vi "AgilentDMM.vi"(4 "error in":T15, 7 "Command":T16) -> (0 "error out":T15, 3 "Response":T13)   [LabVIEW 2018]
uses:
  MOKO_LabViewLibrary/MokoLowLevel/MokoLowLovelControl/MLLC_Command.ctl
  MOKO_LabViewLibrary/MokoLowLevel/MokoLowLovelControl/MLLC_Error.ctl
  MOKO_LabViewLibrary/MokoLowLevel/MokoLowLovelControl/MLLC_Mode.ctl
  MOKO_LabViewLibrary/MokoLowLevel/MokoLowLovelControl/MLLC_Response.ctl
  MOKO_LabViewLibrary/MokoLowLevel/MokoLowLovelControl/MLLC_DriverName.ctl
  MOKO_LabViewLibrary/MokoLowLevel/MokoLowLovelControl/MLLC_Request.ctl
  MOKO_LabViewLibrary/MokoLowLevel/MokoLowLovelControl/MLLC_ErrorCode.ctl
  MOKO_LabViewLibrary/MokoLowLevel/MokoLowLovelControl/MLLC_ResponseInit.ctl
  MOKO_LabViewLibrary/MokoLowLevel/MokoLowLovelControl/MLLC_ConnectCluster.ctl
  MOKO_LabViewLibrary/MokoLowLevel/MokoLowLovelControl/MLLC_InterfaceType.ctl
  MOKO_LabViewLibrary/MokoLowLevel/MokoLowLovelControl/MLLC_OpenedSession.ctl
  MOKO_LabViewLibrary/MokoLowLevel/MokoLowLovelControl/MLLC_InterfaceSettings.ctl
  MOKO_LabViewLibrary/MokoLowLevel/MokoLowLovelControl/MLLC_InterfaceKind.ctl
  data/AgilentDMM_Functions.ctl
  data/AgilentDMM_Models.ctl
panel:
  in  "Settings":T9={"Saved Data"=variant, "Data"={"Connect"={"InterfaceType"=enum."VISA", "OpenedSession"="", "InterfaceSettings"={"Interface"=enum."GPIB", "EOS 4 read"=enum."LF (\\n)", "EOS 4 write"=enum."LF (\\n)", "TMO, ms"=5000, "Sett"=variant(cluster{"Baud Rate":u32, "Data Bits":u16, "Parity":u16, "Stop Bits":u16, "Flow Control":u16, "Eho":bool} {"Baud Rate"=75, "Data Bits"=0, "Parity"=0, "Stop Bits"=0, "Flow Control"=0, "Eho"=FALSE})}}, "Channel"=1, "Func"=enum."VDC", "Model"=enum."L4411"}}
  in  "Response Init array":T10[](array[typedef])=["34401", "34405", "34410", "34411", "34420", "34450", "34461", "34465", "34470", "34475", "U2741"]
  in  "Error Code":T6=5475
  in  "Request":T11="*idn?"
  in  "Driver Name":T12="AgilentDMM"
  in  "Mode":T14=enum."Check"
  # "AgilentDMM"
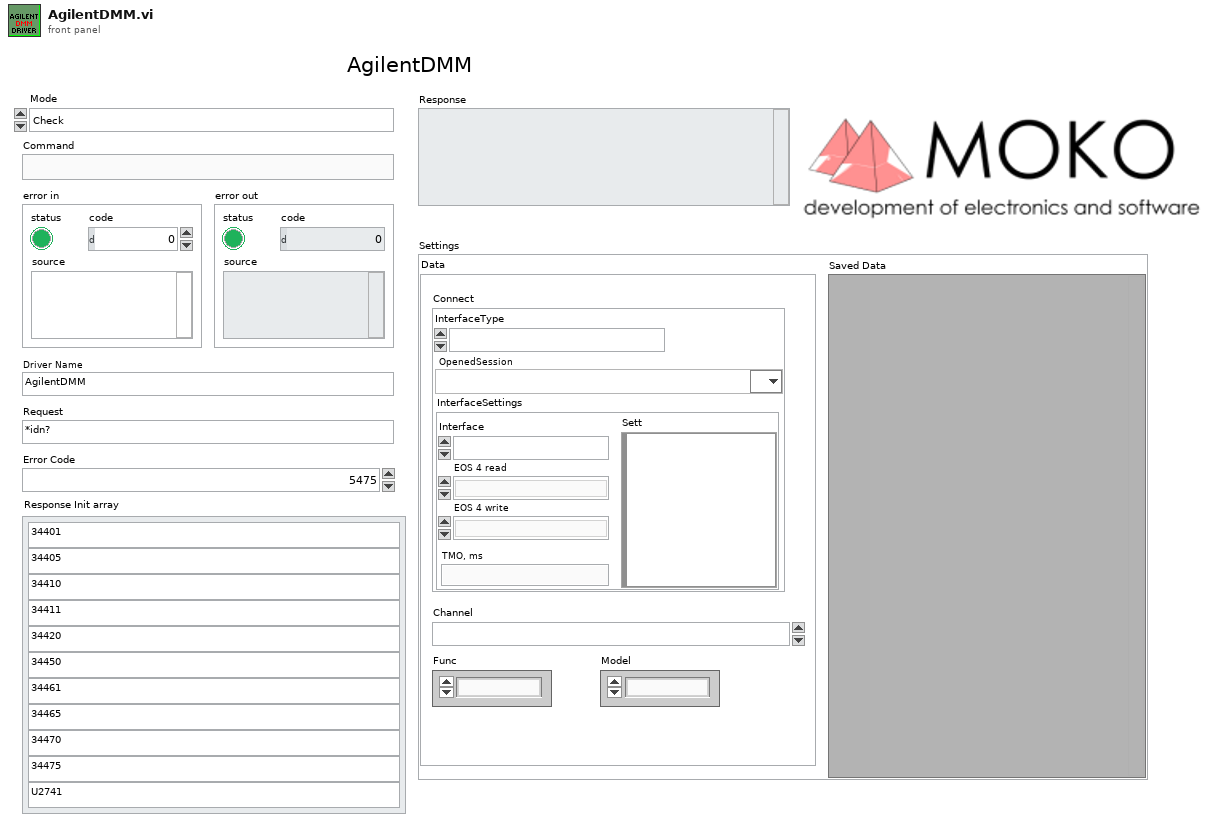
[diagram p1: front panel]
types:
  T1 = typedef "MLLC_ConnectCluster.ctl" = cluster{"InterfaceType":T2, "OpenedSession":T3, "InterfaceSettings":T4}
  T2 = typedef "MLLC_InterfaceType.ctl" = enum16{"VISA", "Prologix USB-GPIB"}
  T3 = typedef "MLLC_OpenedSession.ctl" = refnum<visa-resource-name>
  T4 = typedef "MLLC_InterfaceSettings.ctl" = cluster{"Interface":T5, "EOS 4 read":enum16{"Default (=EOS 4 write)", "CR (\\r)", "LF (\\n)", "None"}, "EOS 4 write":enum16{"CR+LF (\\r\\n)", "CR (\\r)", "LF (\\n)", "None"}, "TMO, ms":i32, "Sett":variant}
  T5 = typedef "MLLC_InterfaceKind.ctl" = enum16{"RS232", "GPIB", "USB", "Ethernet", "another"}
  T6 = typedef "MLLC_ErrorCode.ctl" = u32
  T7 = typedef "AgilentDMM_Functions.ctl" = enum16{"VDC", "VAC", "IDC", "IAC", "F", "R2", "R4", "CAP"}
  T8 = typedef "AgilentDMM_Models.ctl" = enum16{"34401", "34461", "34410", "34411", "34420", "34450", "34405", "U2741", "34470", "34465", "34460", "L4411"}
  T9 = cluster{"Saved Data":variant, "Data":cluster{"Connect":T1, "Channel":T6, "Func":T7, "Model":T8}}
  T10 = typedef "MLLC_ResponseInit.ctl" = string
  T11 = typedef "MLLC_Request.ctl" = string
  T12 = typedef "MLLC_DriverName.ctl" = string
  T13 = typedef "MLLC_Response.ctl" = string
  T14 = typedef "MLLC_Mode.ctl" = enum16{"get", "set", "close", "Init", "Check"}
  T15 = typedef "MLLC_Error.ctl" = errorcluster
  T16 = typedef "MLLC_Command.ctl" = string
  T17 = cluster{"Connect":T1, "Channel":T6, "Func":T7, "Model":T8}
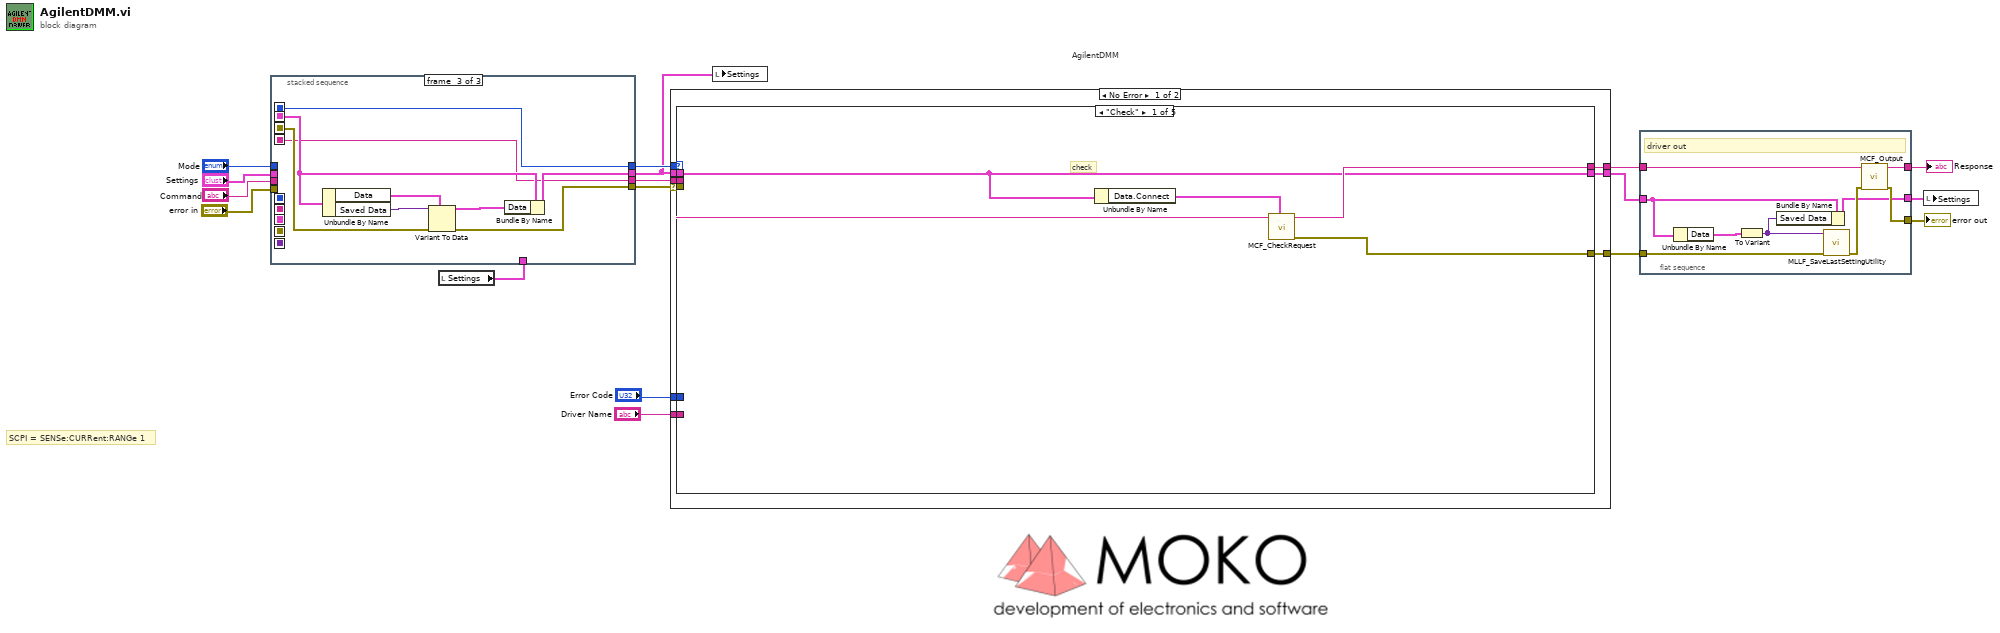
[diagram p0: block diagram]
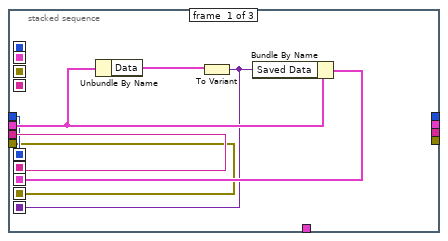
[diagram p2: hidden frame]
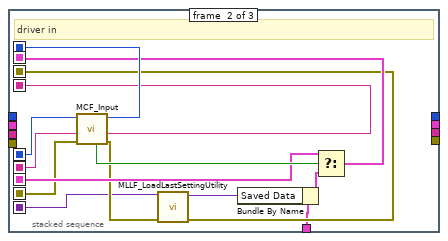
[diagram p3: hidden frame]
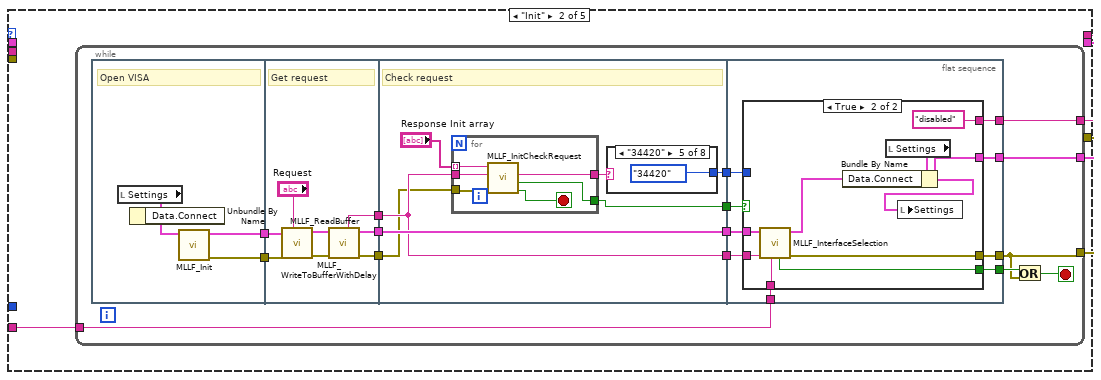
[diagram p4: hidden frame]
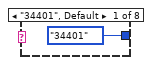
[diagram p5: hidden frame]
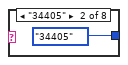
[diagram p6: hidden frame]
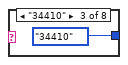
[diagram p7: hidden frame]
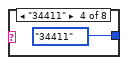
[diagram p8: hidden frame]
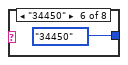
[diagram p9: hidden frame]
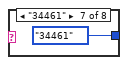
[diagram p10: hidden frame]
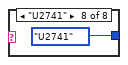
[diagram p11: hidden frame]
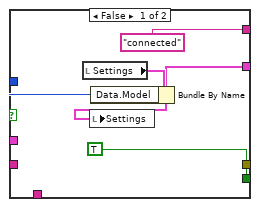
[diagram p12: hidden frame]
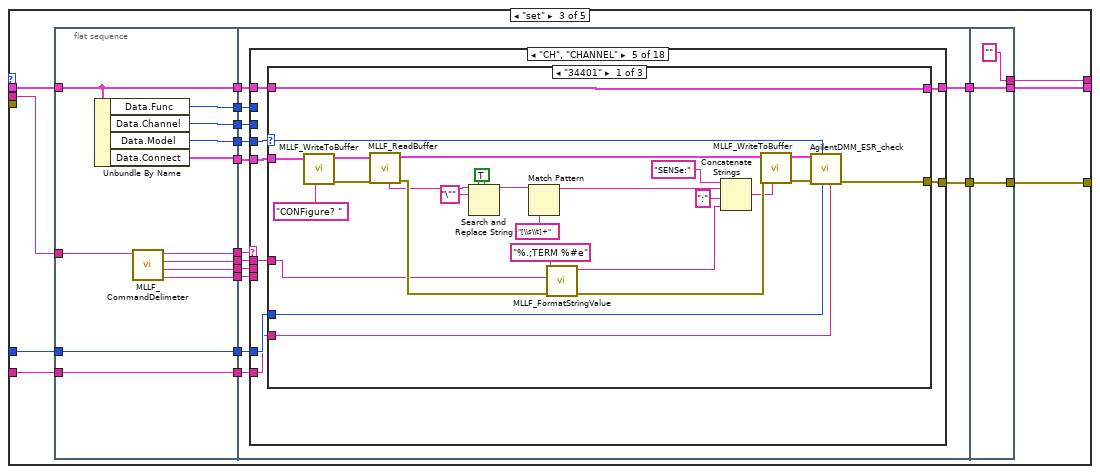
[diagram p13: hidden frame]
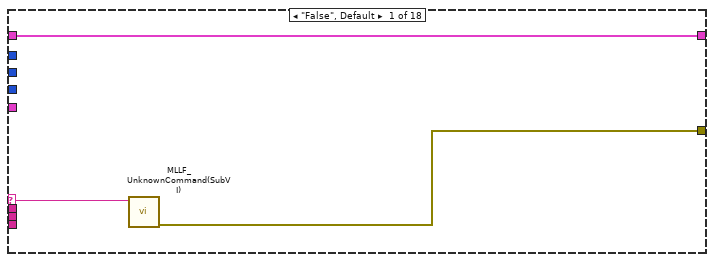
[diagram p14: hidden frame]
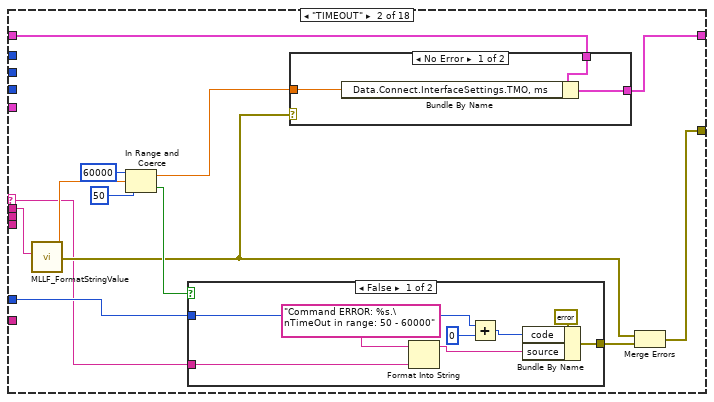
[diagram p15: hidden frame]
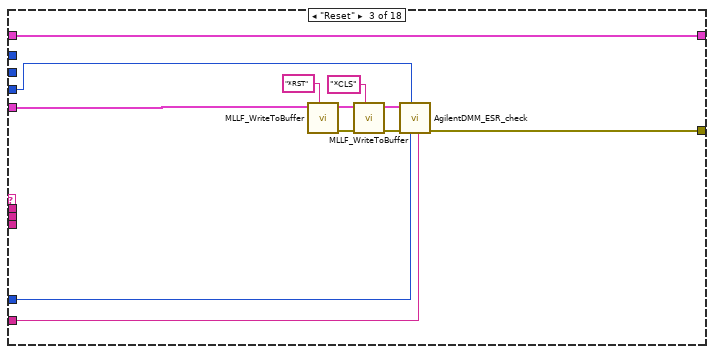
[diagram p18: hidden frame]
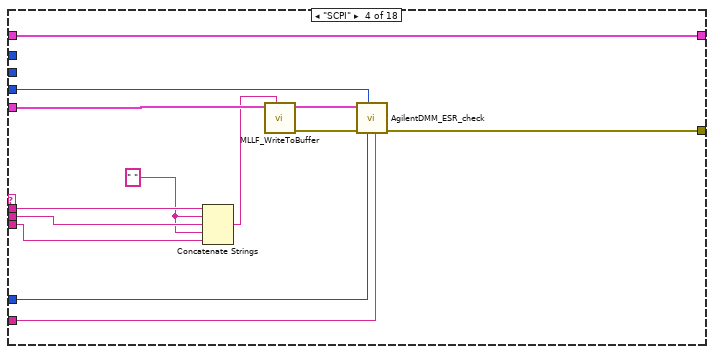
[diagram p19: hidden frame]
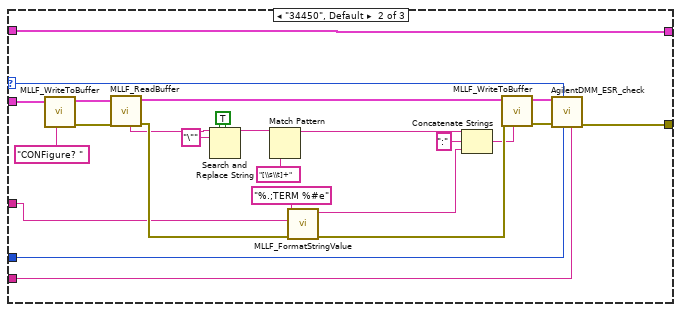
[diagram p20: hidden frame]
diagram:
  # "SCPI = SENSe:CURRent:RANGe 1"
  # "AgilentDMM"
  n1 = local read "Settings"() -> (w8:T9)
  n2 = stacked-sequence {
    seq-local: [w20 _ _] -> [_ w36 _]
    seq-local: [w19 _ _] -> [_ w37 _]
    seq-local: [w22 _ _] -> [_ w32 _]
    seq-local: [w18 _ _] -> [_ w31 _]
    seq-local: [w21 _ _] -> [_ w27 _]
    seq-local: [_ w28 _] -> [_ _ w44]
    seq-local: [_ w38 _] -> [_ _ w41]
    seq-local: [_ w35 _] -> [_ _ w40]
    seq-local: [_ w34 _] -> [_ _ w45]
    tunnel: "Command" -> [w20 _ _]
    tunnel: "Mode" -> [w19 _ _]
    tunnel: "error in" -> [w18 _ _]
    tunnel: "Settings" -> [w23 _ _]
    tunnel: w8 -> [_ w26 _]
    tunnel: [_ _ w40] -> w10
    tunnel: [_ _ w43] -> w1
    tunnel: [_ _ w42] -> w9
    tunnel: [_ _ w41] -> w11
    frame #0 {
      n3 = Unbundle By Name(w23) -> ("Data"=w24:T17)
      n4 = To Variant(anything=w24) -> (Variant=w21:variant)
      n5 = Bundle By Name(cluster=w23, "Saved Data"=w21) -> (w22:T9)
    }
    frame #1 {
      # "driver in"
      n6 = call "MCF_Input.vi"("Error In"=w31, "Command in"=w36, "Mode in"=w37) -> ("Error Out"=w30:errorcluster, "Command out"=w35:string, "Mode out"=w38:T14, "Boolean"=w33:bool)  [unwired: 5 in]
      n7 = call "MLLF_LoadLastSettingUtility.vi"("Error In"=w30, "Save data in"=w27) -> ("Error Out"=w28:errorcluster, "Save data out"=w25:variant)  [unwired: 8 in]
      n8 = Bundle By Name(cluster=w26, "Saved Data"=w25) -> (w29:T9)
      n9 = Select(t=w32, s=w33, f=w29) -> (s? t:f=w34:T9)
    }
    frame #2 {
      n10 = Unbundle By Name(w45) -> ("Data"=w46:T17, "Saved Data"=w39:variant)
      n11 = Variant To Data(error in=w44, type=w46, Variant=w39) -> (data=w47:T17, error out=w42:errorcluster)
      n12 = Bundle By Name(cluster=w45, "Data"=w47) -> (w43:T9)
    }
  }
  n13 = case shown="No Error" w9 {
    selector: w9 -> [w53 w1079]
    tunnel: [w54 w1079] -> w5
    tunnel: w11 -> [w56 _]
    tunnel: [w55 "An error occurred in the driver input module." ("String")] -> w7
    tunnel: w10 -> [w48 _]
    tunnel: w1 -> [w49 w1078]
    tunnel: "Error Code" -> [w52 _]
    tunnel: "Driver Name" -> [w51 _]
    tunnel: [w50 w1078] -> w6
    frame No Error {
      n14 = case shown="\"Check\"" w56 {
        tunnel: [w60 w65 w150 w881 "" ("String")] -> w55
        tunnel: [w61 w63 w153 w882 w1075] -> w54
        tunnel: w53 -> [_ _ _ w899 _]
        tunnel: w52 -> [_ _ w156 w901 _]
        tunnel: w51 -> [w59 w62 w154 w900 _]
        tunnel: [w58 w64 w155 w902 w1074] -> w50
        tunnel: w49 -> [w58 _ w138 w889 w1074]
        tunnel: w48 -> [_ _ w137 w888 _]
        frame "Check" {
          # "check"
          n15 = Unbundle By Name(w58) -> ("Data.Connect"=w57:T1)
          n16 = call "MCF_CheckRequest.vi"("Permanent data.Connect"=w57, "Driver Name"=w59) -> ("Error Out"=w61:errorcluster, "Output String"=w60:string)  [unwired: 8 in]
        }
        frame "Init" {
          n17 = while {
            tunnel: [w68] -> w63
            tunnel: [w67] -> w65
            tunnel: [w66] -> w64
            tunnel: w62 -> [w70]
            stop <- w80 stop-if-true
            n18 = flat-sequence {
              tunnel: [w84] -> w79
              tunnel: [w83] -> w78
              tunnel: w79 -> [w89]
              tunnel: w78 -> [w88]
              tunnel: [w87] -> w77
              tunnel: [w86] -> w76
              tunnel: [w85] -> w75
              tunnel: w77 -> [w95]
              tunnel: w76 -> [w99]
              tunnel: w75 -> [w98]
              tunnel: [w99] -> w74
              tunnel: [w98] -> w73
              tunnel: [w94] -> w72
              tunnel: [w93] -> w71
              tunnel: w74 -> [w121]
              tunnel: w73 -> [w119]
              tunnel: w72 -> [w122]
              tunnel: w71 -> [w120]
              tunnel: w70 -> [w118]
              tunnel: [w117] -> w69
              tunnel: [w116] -> w68
              tunnel: [w115] -> w67
              tunnel: [w114] -> w66
              frame #0 {
                # "Open VISA"
                n19 = local read "Settings"() -> (w82:T9)
                n20 = Unbundle By Name(w82) -> ("Data.Connect"=w81:T1)
                n21 = call "MLLF_Init.vi"("DriverConnect in"=w81) -> ("Error Out"=w84:errorcluster, "DriverConnect out"=w83:T1)  [unwired: 7 in]
              }
              frame #1 {
                # "Get request"
                n22 = call "MLLF_WriteToBufferWithDelay.vi"("Command"="Request", "Error In"=w89, "DriverConnect in"=w88) -> ("Error Out"=w91:errorcluster, "DriverConnect out"=w92:T1)  [unwired: 7 in]
                n23 = call "MLLF_ReadBuffer.vi"("Error In"=w91, "DriverConnect in"=w92) -> ("Error Out"=w87:errorcluster, "DriverConnect out"=w86:T1, "String"=w85:string)  [unwired: 6 in]
              }
              frame #2 {
                # "Check request"
                n24 = for {
                  tunnel: [w102] -> w96
                  tunnel: w98 -> [w104]
                  tunnel: "Response Init array" -> [w105] mode=indexing
                  tunnel: w95 -> [w103]
                  tunnel: [w100] -> w94
                  stop <- w101 stop-if-true
                  n25 = call "MLLF_InitCheckRequest.vi"("error in (no error)"=w103, "Answer"=w104, "Response Init"=w105) -> ("Design ARRAY STOP?"=w101:bool, "Design Interf ARRAY?"=w100:bool, "ResponseInit out"=w102:string)  [unwired: 5 in, 1 out]
                }
                n26 = case shown="\"34420\"" w96 {
                  tunnel: [AgilentDMM_Models."34401" ("Model") AgilentDMM_Models."34405" ("Model") AgilentDMM_Models."34410" ("Model") AgilentDMM_Models."34411" ("Model") AgilentDMM_Models."34420" ("Model") AgilentDMM_Models."34450" ("Model") AgilentDMM_Models."34461" ("Model") AgilentDMM_Models."U2741" ("Model")] -> w93
                  frame "34401", Default {
                  }
                  frame "34405" {
                  }
                  frame "34410" {
                  }
                  frame "34411" {
                  }
                  frame "34420" {
                  }
                  frame "34450" {
                  }
                  frame "34461" {
                  }
                  frame "U2741" {
                  }
                }
              }
              frame #3 {
                n27 = case shown="True" w122 {
                  tunnel: w121 -> [_ w135]
                  tunnel: [TRUE w130] -> w117
                  tunnel: [_ w133] -> w116
                  tunnel: w120 -> [w125 _]
                  tunnel: ["connected" "disabled"] -> w115
                  tunnel: [w123 w131] -> w114
                  tunnel: w119 -> [_ w128]
                  tunnel: w118 -> [_ w129]
                  frame False {
                    n28 = local read "Settings"() -> (w126:T9)
                    n29 = Bundle By Name(cluster=w126, "Data.Model"=w125) -> (w123:T9)
                    n30 = local write "Settings"(w123) -> ()
                  }
                  frame True {
                    n31 = call "MLLF_InterfaceSelection.vi"("Driver Name"=w129, "Answer:"=w128, "DriverConnect in"=w135) -> ("error out"=w133:T15, "DriverConnect out"=w134:T1, "stop init?"=w130:bool)  [unwired: 4 in, 2 out]
                    n32 = local read "Settings"() -> (w136:T9)
                    n33 = Bundle By Name(cluster=w136, "Data.Connect"=w134) -> (w131:T9)
                    n34 = local write "Settings"(w131) -> ()
                  }
                }
              }
            }
            n35 = Or(x=w69, y=w68) -> (x .or. y?=w80:bool)
          }
        }
        frame "set" {
          n36 = flat-sequence {
            tunnel: w154 -> [w167]
            tunnel: w138 -> [w157]
            tunnel: w156 -> [w168]
            tunnel: [w168] -> w149
            tunnel: [w157] -> w148
            tunnel: [w167] -> w147
            tunnel: [w163] -> w146
            tunnel: [w164] -> w145
            tunnel: [w165] -> w144
            tunnel: [w166] -> w143
            tunnel: [w158] -> w142
            tunnel: [w159] -> w141
            tunnel: [w160] -> w140
            tunnel: [w161] -> w139
            tunnel: w137 -> [w162]
            tunnel: [w179] -> w152
            tunnel: [w171] -> w151
            tunnel: w149 -> [w181]
            tunnel: w148 -> [w180]
            tunnel: w147 -> [w178]
            tunnel: w146 -> [w177]
            tunnel: w145 -> [w176]
            tunnel: w144 -> [w175]
            tunnel: w143 -> [w174]
            tunnel: w142 -> [w173]
            tunnel: w141 -> [w172]
            tunnel: w140 -> [w170]
            tunnel: w139 -> [w169]
            tunnel: [w879] -> w153
            tunnel: [w880] -> w155
            tunnel: w152 -> [w880]
            tunnel: w151 -> [w879]
            tunnel: ["" ("String")] -> w150
            frame #0 {
              n37 = Unbundle By Name(w157) -> ("Data.Func"=w166:T7, "Data.Channel"=w165:T6, "Data.Model"=w164:T8, "Data.Connect"=w163:T1)
              n38 = call "MLLF_CommandDelimeter.vi"("command with param"=w162) -> ("param 3"=w161:string, "param 2"=w160:string, "param 1"=w159:string, "command"=w158:string)  [unwired: 6 in, 1 out]
            }
            frame #1 {
              n39 = case shown="\"CH\", \"CHANNEL\"" w173 {
                selector: w173 -> [w183 w186 _ _ _ _ w321 _ _ _ _ _ _ w735 w796 w823 w850 w864]
                tunnel: w172 -> [_ w185 _ w226 w235 _ w322 w397 _ w474 w545 w577 w653 w736 w797 w824 w851 w865]
                tunnel: [w182 w191 w212 w231 w238 _ w328 w401 _ w478 w564 w581 w657 w740 w819 w846 w860 w871] -> w171
                tunnel: w181 -> [_ w192 w214 w233 w241 _ w330 w400 _ w477 w563 w580 w656 w737 w801 w828 w855 w873]
                tunnel: w180 -> [w184 w196 w221 w234 w242 w320 w324 w402 w472 w479 w565 w582 w658 w741 w820 w847 w861 w877]
                tunnel: [w184 w197 w221 w234 w237 w320 w323 w402 w472 w479 w565 w582 w658 w741 w820 w847 w861 w877] -> w179
                tunnel: w177 -> [_ _ w210 w229 w239 _ w327 w398 _ w475 w560 w578 w654 w739 w817 w844 w853 w869]
                tunnel: w178 -> [_ _ w213 w232 w240 _ w329 w399 _ w476 w562 w579 w655 w738 w802 w829 w856 w872]
                tunnel: w176 -> [_ _ w211 w230 w236 _ w326 w396 _ w473 w561 w576 w652 w734 w818 w845 w859 w876]
                tunnel: w175 -> [_ _ _ _ _ _ w325 _ _ _ _ _ _ _ _ _ _ _]
                tunnel: w174 -> [_ _ _ _ _ _ _ _ _ _ _ _ _ _ _ _ _ _]
                tunnel: w170 -> [_ _ _ w225 _ _ _ _ _ _ _ _ _ _ _ _ _ _]
                tunnel: w169 -> [_ _ _ w224 _ _ _ _ _ _ _ _ _ _ _ _ _ _]
                frame "False", Default {
                  n40 = call "MLLF_UnknownCommand(SubVI).vi"("Unknown command"=w183) -> ("error out"=w182:errorcluster)  [unwired: 10 in]
                }
                frame "TIMEOUT" {
                  n41 = call "MLLF_FormatStringValue.vi"("String Value"=w185) -> ("error out"=w187:T15, "number"=w188:dbl)  [unwired: 8 in, 1 out]
                  n42 = In Range and Coerce(upper limit=60000, x=w188, lower limit=50) -> (coerced(x)=w193:dbl, In Range?=w189:bool)
                  n43 = case shown="False" w189 {
                    tunnel: [w204 _] -> w190
                    tunnel: w192 -> [w203 _]
                    tunnel: w186 -> [w202 _]
                    frame False {
                      n44 = Format Into String(format string="Command ERROR: %s.\nTimeOut in range: 50 - 60000", w202) -> (resulting string=w206:string)  [unwired: 2 in, 1 out]
                      n45 = Add(x=w203, y=0) -> (x+y=w207:T6)
                      n46 = Bundle By Name(cluster=errorcluster {"status"=TRUE, "code"=0, "source"=""} ("error out"), "code"=w207, "source"=w206) -> (w204:errorcluster)
                    }
                    frame True {
                    }
                  }
                  n47 = case shown="No Error" w187 {
                    tunnel: [w200 w201] -> w197
                    tunnel: w196 -> [w199 w201]
                    tunnel: w193 -> [w198 _]
                    frame No Error {
                      n48 = Bundle By Name(cluster=w199, "Data.Connect.InterfaceSettings.TMO, ms"=w198) -> (w200:T9)
                    }
                    frame Error {
                    }
                  }
                  n49 = Merge Errors(w187, w190) -> (w191:errorcluster)
                }
                frame "Reset" {
                  n50 = call "MLLF_WriteToBuffer.vi"("String"="*RST", "DriverConnect in"=w210) -> ("error out"=w219:T15, "DriverConnect out"=w220:T1)  [unwired: 6 in]
                  n51 = call "MLLF_WriteToBuffer.vi"("String"="*CLS" ("write buffer"), "error in"=w219, "DriverConnect in"=w220) -> ("error out"=w216:T15, "DriverConnect out"=w215:T1)  [unwired: 5 in]
                  n52 = call "AgilentDMM_ESR_check.vi"("Driver Name"=w213, "Error Code"=w214, "Model"=w211, "error in"=w216, "DriverConnect in"=w215) -> ("error out"=w212:T15)  [unwired: 5 in, 1 out]
                }
                frame "SCPI" {
                  w223 = " " ("string")
                  n53 = Concatenate Strings(w226, w223, w225, w223, w224) -> (w222:string)
                  n54 = call "MLLF_WriteToBuffer.vi"("String"=w222, "DriverConnect in"=w229) -> ("error out"=w227:T15, "DriverConnect out"=w228:T1)  [unwired: 6 in]
                  n55 = call "AgilentDMM_ESR_check.vi"("Driver Name"=w232, "Error Code"=w233, "Model"=w230, "error in"=w227, "DriverConnect in"=w228) -> ("error out"=w231:T15)  [unwired: 5 in, 1 out]
                }
                frame "CH", "CHANNEL" {
                  n56 = case shown="\"34401\"" w236 {
                    selector: w236 -> [w245 w270 w296]
                    tunnel: w242 -> [w247 w272 w301]
                    tunnel: w241 -> [w249 w274 w300]
                    tunnel: w240 -> [w248 w273 w295]
                    tunnel: w239 -> [w246 w271 w299]
                    tunnel: [w250 w275 w298] -> w238
                    tunnel: [w247 w272 w297] -> w237
                    tunnel: w235 -> [w244 w269 w294]
                    frame "34401" {
                      w254 = TRUE ("replace all? (F)")
                      n57 = call "MLLF_WriteToBuffer.vi"("String"="CONFigure? ", "DriverConnect in"=w246) -> ("error out"=w263:T15, "DriverConnect out"=w264:T1)  [unwired: 6 in]
                      n58 = call "MLLF_ReadBuffer.vi"("Error In"=w263, "DriverConnect in"=w264) -> ("Error Out"=w262:errorcluster, "DriverConnect out"=w261:T1, "String"=w256:string)  [unwired: 6 in]
                      n59 = Search and Replace String(replace all?=w254, case sensitive?=w254, input string=w256, search string="\"") -> (result string=w255:string)  [unwired: 4 in, 3 out]
                      n60 = Match Pattern(string=w255, regular expression="[\\s\\t]+") -> (before substring=w257:string)  [unwired: 1 in, 3 out]
                      n61 = call "MLLF_FormatStringValue.vi"("error in"=w262, "String Value"=w244, "Format"="%.;TERM %#e" ("format string")) -> ("error out"=w268:T15, "String Value Formated"=w259:T16)  [unwired: 6 in, 1 out]
                      n62 = Concatenate Strings("SENSe:" ("string"), w257, ":" ("string"), w259) -> (w252:string)
                      n63 = call "MLLF_WriteToBuffer.vi"("String"=w252, "error in"=w268, "DriverConnect in"=w261) -> ("error out"=w267:T15, "DriverConnect out"=w266:T1)  [unwired: 5 in]
                      n64 = call "AgilentDMM_ESR_check.vi"("Driver Name"=w248, "Error Code"=w249, "Model"=w245, "error in"=w267, "DriverConnect in"=w266) -> ("error out"=w250:T15)  [unwired: 5 in, 1 out]
                    }
                    frame "34450", Default {
                      w279 = TRUE ("replace all? (F)")
                      n65 = call "MLLF_WriteToBuffer.vi"("String"="CONFigure? ", "DriverConnect in"=w271) -> ("error out"=w288:T15, "DriverConnect out"=w289:T1)  [unwired: 6 in]
                      n66 = call "MLLF_ReadBuffer.vi"("Error In"=w288, "DriverConnect in"=w289) -> ("Error Out"=w287:errorcluster, "DriverConnect out"=w286:T1, "String"=w281:string)  [unwired: 6 in]
                      n67 = Search and Replace String(replace all?=w279, case sensitive?=w279, input string=w281, search string="\"") -> (result string=w280:string)  [unwired: 4 in, 3 out]
                      n68 = Match Pattern(string=w280, regular expression="[\\s\\t]+") -> (before substring=w282:string)  [unwired: 1 in, 3 out]
                      n69 = call "MLLF_FormatStringValue.vi"("error in"=w287, "String Value"=w269, "Format"="%.;TERM %#e" ("format string")) -> ("error out"=w293:T15, "String Value Formated"=w284:T16)  [unwired: 6 in, 1 out]
                      n70 = Concatenate Strings(w282, ":" ("string"), w284) -> (w277:string)
                      n71 = call "MLLF_WriteToBuffer.vi"("String"=w277, "error in"=w293, "DriverConnect in"=w286) -> ("error out"=w292:T15, "DriverConnect out"=w291:T1)  [unwired: 5 in]
                      n72 = call "AgilentDMM_ESR_check.vi"("Driver Name"=w273, "Error Code"=w274, "Model"=w270, "error in"=w292, "DriverConnect in"=w291) -> ("error out"=w275:T15)  [unwired: 5 in, 1 out]
                    }
                    frame "34420" {
                      n73 = call "MLLF_FormatStringValue.vi"("String Value"=w294, "Format"="%d" ("format")) -> ("error out"=w313:T15, "String Value Formated"=w306:T16)  [unwired: 7 in, 1 out]
                      n74 = call "MLLF_ParameterSelect.vi"("Command to equipment"=string[] ["1", "2"] ("Parameters"), "Names"=string[][] [["1"], ["2"]], "Input"=w306, "Error In"=w313, "Command"=w294, "Driver Name"=w295, "Error Code"=w300) -> ("Choice"=w303:string, "Error Out"=w305:errorcluster)  [unwired: 7 in]
                      n75 = call "MLLF_ParameterSelect.vi"("Command to equipment"=string[] ["ROUTe:TERMinals FRONt1", "ROUTe:TERMinals FRONt2"] ("Names"), "Names"=string[][] [["1"], ["2"]], "Input"=w306, "Error In"=w305, "Command"=w294, "Driver Name"=w295, "Error Code"=w300) -> ("Choice"=w309:string, "Error Out"=w308:errorcluster)  [unwired: 7 in]
                      n76 = call "MLLF_WriteToBuffer.vi"("String"=w309, "error in"=w308, "DriverConnect in"=w299) -> ("error out"=w304:T15, "DriverConnect out"=w307:T1)  [unwired: 5 in]
                      n77 = call "AgilentDMM_ESR_check.vi"("Driver Name"=w295, "Error Code"=w300, "Model"=w296, "error in"=w304, "DriverConnect in"=w307) -> ("error out"=w298:T15)  [unwired: 5 in, 1 out]
                      n78 = Decimal String To Number(string=w303) -> (number=w302:i32)  [unwired: 2 in, 1 out]
                      n79 = case shown="No Error" w298 {
                        tunnel: [w318 w319] -> w297
                        tunnel: w301 -> [w317 w319]
                        tunnel: w302 -> [w316 _]
                        frame No Error {
                          n80 = Bundle By Name(cluster=w317, "Data.Channel"=w316) -> (w318:T9)
                        }
                        frame Error {
                        }
                      }
                    }
                  }
                }
                frame "<----MAIN FUNCTIONS---->" {
                }
                frame "Func", "Function" {
                  # "FUNC=VDC"
                  n81 = case shown="Default" w326 {
                    selector: w326 -> [w357 w379]
                    tunnel: w322 -> [w356 w368]
                    tunnel: w330 -> [w363 w383]
                    tunnel: w329 -> [w362 w382]
                    tunnel: [w361 w381] -> w328
                    tunnel: w327 -> [w359 w380]
                    tunnel: w325 -> [_ w374]
                    tunnel: w321 -> [w355 _]
                    frame Default {
                      n82 = call "MLLF_ParameterSelect.vi"("Command to equipment"=string[] ["CONF:VOLT:DC auto", "CONF:VOLT:AC auto", "CONF:CURR:DC auto", "CONF:CURR:AC auto", "CONF:RES auto", "CONF:FRES auto", "CONF:FREQ", "CONF:TC", "CONF:PER", "CONF:TEMP", "CONF:CAP auto"] ("Names"), "Names"=string[][] [["VDC", "", ""], ["VAC", "", ""], ["IDC", "", ""], ["IAC", "", ""], ["R", "R2", "R2WIRE"], ["R4", "R4WIRE", ""], ["F", "", ""], ["TC", "", ""], ["P", "Period", ""], ["RTD", "PRT", ""], ["C", "CAP", ""]], "Input"=w356, "Command"=w355, "Driver Name"=w362, "Error Code"=w363) -> ("Choice"=w358:string, "Error Out"=w360:errorcluster)  [unwired: 8 in]
                      n83 = call "MLLF_WriteToBuffer.vi"("String"=w358, "error in"=w360, "DriverConnect in"=w359) -> ("error out"=w367:T15, "DriverConnect out"=w366:T1)  [unwired: 5 in]
                      n84 = call "AgilentDMM_ESR_check.vi"("Driver Name"=w362, "Error Code"=w363, "Model"=w357, "error in"=w367, "DriverConnect in"=w366) -> ("error out"=w361:T15)  [unwired: 5 in, 1 out]
                    }
                    frame "34420" {
                      n85 = Equal?(x=u8 1 ("y"), y=w374) -> (x = y?=w376:bool)
                      n86 = Select(t="ROUTe:TERMinals FRONt1" ("String"), s=w376, f="ROUTe:TERMinals FRONt2" ("String")) -> (s? t:f=w370:string)
                      n87 = call "MLLF_ParameterSelect.vi"("Command to equipment"=string[] ["CONF:VOLT:DC auto", "CONF:RES auto", "CONF:FRES auto", "CONF:TC", "CONF:TEMP"] ("Names"), "Names"=string[][] [["VDC", "", ""], ["R", "R2", "R2WIRE"], ["R4", "R4WIRE", ""], ["TC", "", ""], ["RTD", "PRT", ""]], "Input"=w368, "Command"=w368, "Driver Name"=w382, "Error Code"=w383) -> ("Choice"=w369:string, "Error Out"=w371:errorcluster)  [unwired: 8 in]
                      n88 = case shown="\"True\", Default" w369 {
                        selector: w369 -> [w388 w390]
                        tunnel: [w388 w394] -> w373
                        tunnel: [w389 w393] -> w372
                        tunnel: w371 -> [w389 w392]
                        tunnel: w370 -> [_ w391]
                        frame "False" {
                        }
                        frame "True", Default {
                          n89 = Format Into String(format string="%S\n%S", error in=w392, w390, w391) -> (resulting string=w394:string, error out=w393:errorcluster)  [unwired: 1 in]
                        }
                      }
                      n90 = call "MLLF_WriteToBuffer.vi"("String"=w373, "error in"=w372, "DriverConnect in"=w380) -> ("error out"=w387:T15, "DriverConnect out"=w386:T1)  [unwired: 5 in]
                      n91 = call "AgilentDMM_ESR_check.vi"("Driver Name"=w382, "Error Code"=w383, "Model"=w379, "error in"=w387, "DriverConnect in"=w386) -> ("error out"=w381:T15)  [unwired: 5 in, 1 out]
                    }
                  }
                  n92 = case shown="\"IDC\"" w322 {
                    tunnel: w324 -> [w333 w336 w339 w342 w345 w348 w351 w354]
                    tunnel: [w332 w335 w338 w341 w344 w347 w350 w353] -> w323
                    frame "VDC", Default {
                      n93 = Bundle By Name(cluster=w333, "Data.Func"=AgilentDMM_Functions."VDC" ("Func")) -> (w332:T9)
                    }
                    frame "VAC" {
                      n94 = Bundle By Name(cluster=w336, "Data.Func"=AgilentDMM_Functions."VAC" ("Func")) -> (w335:T9)
                    }
                    frame "IDC" {
                      n95 = Bundle By Name(cluster=w339, "Data.Func"=AgilentDMM_Functions."IDC" ("Func")) -> (w338:T9)
                    }
                    frame "IAC" {
                      n96 = Bundle By Name(cluster=w342, "Data.Func"=AgilentDMM_Functions."IAC" ("Func")) -> (w341:T9)
                    }
                    frame "R", "R2", "R2WI" {
                      n97 = Bundle By Name(cluster=w345, "Data.Func"=AgilentDMM_Functions."R2" ("Func")) -> (w344:T9)
                    }
                    frame "R4", "R4WI" {
                      n98 = Bundle By Name(cluster=w348, "Data.Func"=AgilentDMM_Functions."R4" ("Func")) -> (w347:T9)
                    }
                    frame "F" {
                      n99 = Bundle By Name(cluster=w351, "Data.Func"=AgilentDMM_Functions."F" ("Func")) -> (w350:T9)
                    }
                    frame "C", "CAP" {
                      n100 = Bundle By Name(cluster=w354, "Data.Func"=AgilentDMM_Functions."CAP" ("Func")) -> (w353:T9)
                    }
                  }
                }
                frame "Range" {
                  n101 = case shown="\"34401\"" w396 {
                    tunnel: [w422 w457] -> w401
                    tunnel: w400 -> [w421 w456]
                    tunnel: w399 -> [w420 w455]
                    tunnel: w396 -> [w419 w454]
                    tunnel: w398 -> [w418 w453]
                    tunnel: w397 -> [w404 w439]
                    frame "34461", Default {
                      w407 = TRUE ("replace all? (F)")
                      n102 = call "MLLF_WriteToBuffer.vi"("String"="CONFigure? ", "DriverConnect in"=w418) -> ("error out"=w415:T15, "DriverConnect out"=w416:T1)  [unwired: 6 in]
                      n103 = call "MLLF_ReadBuffer.vi"("Error In"=w415, "DriverConnect in"=w416) -> ("Error Out"=w403:errorcluster, "DriverConnect out"=w414:T1, "String"=w409:string)  [unwired: 6 in]
                      n104 = Search and Replace String(replace all?=w407, case sensitive?=w407, input string=w409, search string="\"") -> (result string=w408:string)  [unwired: 4 in, 3 out]
                      n105 = case shown="\"MIN\"" w404 {
                        selector: w404 -> [w427 _ _ _]
                        tunnel: [w430 w431 w433 w435] -> w425
                        tunnel: [w429 "RANG:AUTO ON" ("String") "RANG MIN" ("String") "RANG MAX" ("String")] -> w412
                        tunnel: w403 -> [w426 w431 w433 w435]
                        frame "False", Default {
                          n106 = call "MLLF_FormatStringValue.vi"("error in"=w426, "String Value"=w427, "Format"="RANG %#e" ("format string")) -> ("error out"=w430:T15, "String Value Formated"=w429:T16)  [unwired: 6 in, 1 out]
                        }
                        frame "Auto" {
                        }
                        frame "MIN" {
                        }
                        frame "MAX" {
                        }
                      }
                      n107 = Match Pattern(string=w408, regular expression="[\\s\\t]+") -> (before substring=w410:string)  [unwired: 1 in, 3 out]
                      n108 = Concatenate Strings(w410, ":" ("string"), w412) -> (w405:string)
                      n109 = call "MLLF_WriteToBuffer.vi"("String"=w405, "error in"=w425, "DriverConnect in"=w414) -> ("error out"=w424:T15, "DriverConnect out"=w423:T1)  [unwired: 5 in]
                      n110 = call "AgilentDMM_ESR_check.vi"("Driver Name"=w420, "Error Code"=w421, "Model"=w419, "error in"=w424, "DriverConnect in"=w423) -> ("error out"=w422:T15)  [unwired: 5 in, 1 out]
                    }
                    frame "34401" {
                      w442 = TRUE ("replace all? (F)")
                      n111 = call "MLLF_WriteToBuffer.vi"("String"="CONFigure? ", "DriverConnect in"=w453) -> ("error out"=w450:T15, "DriverConnect out"=w451:T1)  [unwired: 6 in]
                      n112 = call "MLLF_ReadBuffer.vi"("Error In"=w450, "DriverConnect in"=w451) -> ("Error Out"=w438:errorcluster, "DriverConnect out"=w449:T1, "String"=w444:string)  [unwired: 6 in]
                      n113 = Search and Replace String(replace all?=w442, case sensitive?=w442, input string=w444, search string="\"") -> (result string=w443:string)  [unwired: 4 in, 3 out]
                      n114 = case shown="\"MIN\"" w439 {
                        selector: w439 -> [w462 _ _ _]
                        tunnel: [w465 w466 w468 w470] -> w460
                        tunnel: [w464 "RANG:AUTO ON" ("String") "RANG MIN" ("String") "RANG MAX" ("String")] -> w447
                        tunnel: w438 -> [w461 w466 w468 w470]
                        frame "False", Default {
                          n115 = call "MLLF_FormatStringValue.vi"("error in"=w461, "String Value"=w462, "Format"="RANG %#e" ("format string")) -> ("error out"=w465:T15, "String Value Formated"=w464:T16)  [unwired: 6 in, 1 out]
                        }
                        frame "Auto" {
                        }
                        frame "MIN" {
                        }
                        frame "MAX" {
                        }
                      }
                      n116 = Match Pattern(string=w443, regular expression="[\\s\\t]+") -> (before substring=w445:string)  [unwired: 1 in, 3 out]
                      n117 = Concatenate Strings("SENSe:" ("string"), w445, ":" ("string"), w447) -> (w440:string)
                      n118 = call "MLLF_WriteToBuffer.vi"("String"=w440, "error in"=w460, "DriverConnect in"=w449) -> ("error out"=w459:T15, "DriverConnect out"=w458:T1)  [unwired: 5 in]
                      n119 = call "AgilentDMM_ESR_check.vi"("Driver Name"=w455, "Error Code"=w456, "Model"=w454, "error in"=w459, "DriverConnect in"=w458) -> ("error out"=w457:T15)  [unwired: 5 in, 1 out]
                    }
                  }
                }
                frame "---------ADDITIONAL---------" {
                }
                frame "Res", "Resolution" {
                  n120 = case shown="\"34401\"" w473 {
                    selector: w473 -> [w480 w513]
                    tunnel: [w499 w532] -> w478
                    tunnel: w477 -> [w498 w531]
                    tunnel: w476 -> [w497 w530]
                    tunnel: w475 -> [w496 w529]
                    tunnel: w474 -> [w481 w514]
                    frame "34461", Default {
                      w484 = TRUE ("replace all? (F)")
                      n121 = call "MLLF_WriteToBuffer.vi"("String"="CONFigure? ", "DriverConnect in"=w496) -> ("error out"=w493:T15, "DriverConnect out"=w494:T1)  [unwired: 6 in]
                      n122 = call "MLLF_ReadBuffer.vi"("Error In"=w493, "DriverConnect in"=w494) -> ("Error Out"=w492:errorcluster, "DriverConnect out"=w491:T1, "String"=w486:string)  [unwired: 6 in]
                      n123 = Search and Replace String(replace all?=w484, case sensitive?=w484, input string=w486, search string="\"") -> (result string=w485:string)  [unwired: 4 in, 3 out]
                      n124 = case shown="\"MAX\"" w481 {
                        selector: w481 -> [w504 _ _]
                        tunnel: [w507 w508 w510] -> w502
                        tunnel: [w506 "RES MAX" ("String") "RES MIN" ("String")] -> w489
                        tunnel: w492 -> [w503 w508 w510]
                        frame "False", Default {
                          n125 = call "MLLF_FormatStringValue.vi"("error in"=w503, "String Value"=w504, "Format"="RES %#e" ("format string")) -> ("error out"=w507:T15, "String Value Formated"=w506:T16)  [unwired: 6 in, 1 out]
                        }
                        frame "MAX" {
                        }
                        frame "MIN" {
                        }
                      }
                      n126 = Match Pattern(string=w485, regular expression="[\\s\\t]+") -> (before substring=w487:string)  [unwired: 1 in, 3 out]
                      n127 = Concatenate Strings(w487, ":" ("string"), w489) -> (w482:string)
                      n128 = call "MLLF_WriteToBuffer.vi"("String"=w482, "error in"=w502, "DriverConnect in"=w491) -> ("error out"=w501:T15, "DriverConnect out"=w500:T1)  [unwired: 5 in]
                      n129 = call "AgilentDMM_ESR_check.vi"("Driver Name"=w497, "Error Code"=w498, "Model"=w480, "error in"=w501, "DriverConnect in"=w500) -> ("error out"=w499:T15)  [unwired: 5 in, 1 out]
                    }
                    frame "34401" {
                      w517 = TRUE ("replace all? (F)")
                      n130 = call "MLLF_WriteToBuffer.vi"("String"="CONFigure? ", "DriverConnect in"=w529) -> ("error out"=w526:T15, "DriverConnect out"=w527:T1)  [unwired: 6 in]
                      n131 = call "MLLF_ReadBuffer.vi"("Error In"=w526, "DriverConnect in"=w527) -> ("Error Out"=w525:errorcluster, "DriverConnect out"=w524:T1, "String"=w519:string)  [unwired: 6 in]
                      n132 = Search and Replace String(replace all?=w517, case sensitive?=w517, input string=w519, search string="\"") -> (result string=w518:string)  [unwired: 4 in, 3 out]
                      n133 = case shown="\"MIN\"" w514 {
                        selector: w514 -> [w537 _ _]
                        tunnel: [w540 w541 w543] -> w535
                        tunnel: [w539 "RES MAX" ("String") "RES MIN" ("String")] -> w522
                        tunnel: w525 -> [w536 w541 w543]
                        frame "False", Default {
                          n134 = call "MLLF_FormatStringValue.vi"("error in"=w536, "String Value"=w537, "Format"="RES %#e" ("format string")) -> ("error out"=w540:T15, "String Value Formated"=w539:T16)  [unwired: 6 in, 1 out]
                        }
                        frame "MAX" {
                        }
                        frame "MIN" {
                        }
                      }
                      n135 = Match Pattern(string=w518, regular expression="[\\s\\t]+") -> (before substring=w520:string)  [unwired: 1 in, 3 out]
                      n136 = Concatenate Strings("SENSe:" ("string"), w520, ":" ("string"), w522) -> (w515:string)
                      n137 = call "MLLF_WriteToBuffer.vi"("String"=w515, "error in"=w535, "DriverConnect in"=w524) -> ("error out"=w534:T15, "DriverConnect out"=w533:T1)  [unwired: 5 in]
                      n138 = call "AgilentDMM_ESR_check.vi"("Driver Name"=w530, "Error Code"=w531, "Model"=w513, "error in"=w534, "DriverConnect in"=w533) -> ("error out"=w532:T15)  [unwired: 5 in, 1 out]
                    }
                  }
                }
                frame "Aper", "Aperture", "MeasTime" {
                  w548 = TRUE ("replace all? (F)")
                  n139 = call "MLLF_WriteToBuffer.vi"("String"="CONFigure? ", "DriverConnect in"=w560) -> ("error out"=w557:T15, "DriverConnect out"=w558:T1)  [unwired: 6 in]
                  n140 = call "MLLF_ReadBuffer.vi"("Error In"=w557, "DriverConnect in"=w558) -> ("Error Out"=w556:errorcluster, "DriverConnect out"=w555:T1, "String"=w550:string)  [unwired: 6 in]
                  n141 = Search and Replace String(replace all?=w548, case sensitive?=w548, input string=w550, search string="\"") -> (result string=w549:string)  [unwired: 4 in, 3 out]
                  n142 = case shown="\"OFF\"" w545 {
                    selector: w545 -> [w570 _]
                    tunnel: [w573 w574] -> w568
                    tunnel: [w572 "APER:ENAB OFF" ("String")] -> w553
                    tunnel: w556 -> [w569 w574]
                    frame "False", Default {
                      n143 = call "MLLF_FormatStringValue.vi"("error in"=w569, "String Value"=w570, "Format"="APER %#e" ("format string")) -> ("error out"=w573:T15, "String Value Formated"=w572:T16)  [unwired: 6 in, 1 out]
                    }
                    frame "OFF" {
                    }
                  }
                  n144 = Match Pattern(string=w549, regular expression="[\\s\\t]+") -> (before substring=w551:string)  [unwired: 1 in, 3 out]
                  n145 = Concatenate Strings(w551, ":" ("string"), w553) -> (w546:string)
                  n146 = call "MLLF_WriteToBuffer.vi"("String"=w546, "error in"=w568, "DriverConnect in"=w555) -> ("error out"=w567:T15, "DriverConnect out"=w566:T1)  [unwired: 5 in]
                  n147 = call "AgilentDMM_ESR_check.vi"("Driver Name"=w562, "Error Code"=w563, "Model"=w561, "error in"=w567, "DriverConnect in"=w566) -> ("error out"=w564:T15)  [unwired: 5 in, 1 out]
                }
                frame "IntegrationTime", "IntTime", "NPLC" {
                  n148 = case shown="\"34401\"" w576 {
                    tunnel: [w602 w636] -> w581
                    tunnel: w580 -> [w601 w635]
                    tunnel: w579 -> [w600 w634]
                    tunnel: w576 -> [w599 w633]
                    tunnel: w578 -> [w598 w632]
                    tunnel: w577 -> [w584 w618]
                    frame "34401" {
                      w587 = TRUE ("replace all? (F)")
                      n149 = call "MLLF_WriteToBuffer.vi"("String"="CONFigure? ", "DriverConnect in"=w598) -> ("error out"=w595:T15, "DriverConnect out"=w596:T1)  [unwired: 6 in]
                      n150 = call "MLLF_ReadBuffer.vi"("Error In"=w595, "DriverConnect in"=w596) -> ("DriverConnect out"=w594:T1, "String"=w589:string)  [unwired: 6 in, 1 out]
                      n151 = Search and Replace String(replace all?=w587, case sensitive?=w587, input string=w589, search string="\"") -> (result string=w588:string)  [unwired: 4 in, 3 out]
                      n152 = case shown="\"MIN\"" w584 {
                        tunnel: [w609 w613 w617] -> w605
                        tunnel: [w608 w612 w616] -> w592
                        tunnel: w584 -> [w606 w610 w614]
                        frame Default {
                          n153 = call "MLLF_FormatStringValue.vi"("String Value"=w606, "Format"="NPLC %#e" ("format string")) -> ("error out"=w609:T15, "String Value Formated"=w608:T16)  [unwired: 7 in, 1 out]
                        }
                        frame "MIN" {
                          n154 = call "MLLF_FormatStringValue.vi"("String Value"=w610, "Format"="NPLC MIN" ("format string")) -> ("error out"=w613:T15, "String Value Formated"=w612:T16)  [unwired: 7 in, 1 out]
                        }
                        frame "MAX" {
                          n155 = call "MLLF_FormatStringValue.vi"("String Value"=w614, "Format"="NPLC MAX" ("format string")) -> ("error out"=w617:T15, "String Value Formated"=w616:T16)  [unwired: 7 in, 1 out]
                        }
                      }
                      n156 = Match Pattern(string=w588, regular expression="[\\s\\t]+") -> (before substring=w590:string)  [unwired: 1 in, 3 out]
                      n157 = Concatenate Strings("SENSe:" ("string"), w590, ":" ("string"), w592) -> (w585:string)
                      n158 = call "MLLF_WriteToBuffer.vi"("String"=w585, "error in"=w605, "DriverConnect in"=w594) -> ("error out"=w604:T15, "DriverConnect out"=w603:T1)  [unwired: 5 in]
                      n159 = call "AgilentDMM_ESR_check.vi"("Driver Name"=w600, "Error Code"=w601, "Model"=w599, "error in"=w604, "DriverConnect in"=w603) -> ("error out"=w602:T15)  [unwired: 5 in, 1 out]
                    }
                    frame Default {
                      w621 = TRUE ("replace all? (F)")
                      n160 = call "MLLF_WriteToBuffer.vi"("String"="CONFigure? ", "DriverConnect in"=w632) -> ("error out"=w629:T15, "DriverConnect out"=w630:T1)  [unwired: 6 in]
                      n161 = call "MLLF_ReadBuffer.vi"("Error In"=w629, "DriverConnect in"=w630) -> ("DriverConnect out"=w628:T1, "String"=w623:string)  [unwired: 6 in, 1 out]
                      n162 = Search and Replace String(replace all?=w621, case sensitive?=w621, input string=w623, search string="\"") -> (result string=w622:string)  [unwired: 4 in, 3 out]
                      n163 = case shown="Default" w618 {
                        tunnel: [w643 w647 w651] -> w639
                        tunnel: [w642 w646 w650] -> w626
                        tunnel: w618 -> [w640 w644 w648]
                        frame Default {
                          n164 = call "MLLF_FormatStringValue.vi"("String Value"=w640, "Format"="%.;NPLC %#e" ("format string")) -> ("error out"=w643:T15, "String Value Formated"=w642:T16)  [unwired: 7 in, 1 out]
                        }
                        frame "MIN" {
                          n165 = call "MLLF_FormatStringValue.vi"("String Value"=w644, "Format"="NPLC MIN" ("format string")) -> ("error out"=w647:T15, "String Value Formated"=w646:T16)  [unwired: 7 in, 1 out]
                        }
                        frame "MAX" {
                          n166 = call "MLLF_FormatStringValue.vi"("String Value"=w648, "Format"="NPLC MAX" ("format string")) -> ("error out"=w651:T15, "String Value Formated"=w650:T16)  [unwired: 7 in, 1 out]
                        }
                      }
                      n167 = Match Pattern(string=w622, regular expression="[\\s\\t]+") -> (before substring=w624:string)  [unwired: 1 in, 3 out]
                      n168 = Concatenate Strings(w624, ":" ("string"), w626) -> (w619:string)
                      n169 = call "MLLF_WriteToBuffer.vi"("String"=w619, "error in"=w639, "DriverConnect in"=w628) -> ("error out"=w638:T15, "DriverConnect out"=w637:T1)  [unwired: 5 in]
                      n170 = call "AgilentDMM_ESR_check.vi"("Driver Name"=w634, "Error Code"=w635, "Model"=w633, "error in"=w638, "DriverConnect in"=w637) -> ("error out"=w636:T15)  [unwired: 5 in, 1 out]
                    }
                  }
                }
                frame "ACBand", "ACBandwidth", "Band", "Bandwidth" {
                  n171 = case shown="\"34401\"" w652 {
                    selector: w652 -> [w659 w697]
                    tunnel: [w678 w715] -> w657
                    tunnel: w656 -> [w677 w714]
                    tunnel: w655 -> [w676 w713]
                    tunnel: w654 -> [w675 w712]
                    tunnel: w653 -> [w660 w699]
                    frame "34461", Default {
                      w663 = TRUE ("replace all? (F)")
                      n172 = call "MLLF_WriteToBuffer.vi"("String"="CONFigure? ", "DriverConnect in"=w675) -> ("error out"=w672:T15, "DriverConnect out"=w673:T1)  [unwired: 6 in]
                      n173 = call "MLLF_ReadBuffer.vi"("Error In"=w672, "DriverConnect in"=w673) -> ("Error Out"=w671:errorcluster, "DriverConnect out"=w670:T1, "String"=w665:string)  [unwired: 6 in]
                      n174 = case shown="\"MIN\"" w660 {
                        selector: w660 -> [w682 w687 w692]
                        tunnel: [w686 w691 w696] -> w681
                        tunnel: w671 -> [w685 w690 w695]
                        tunnel: [w684 w689 w694] -> w668
                        frame Default {
                          n175 = call "MLLF_FormatStringValue.vi"("error in"=w685, "String Value"=w682, "Format"="%.;BAND %#f" ("format string")) -> ("error out"=w686:T15, "String Value Formated"=w684:T16)  [unwired: 6 in, 1 out]
                        }
                        frame "MAX" {
                          n176 = call "MLLF_FormatStringValue.vi"("error in"=w690, "String Value"=w687, "Format"="BAND MAX" ("format string")) -> ("error out"=w691:T15, "String Value Formated"=w689:T16)  [unwired: 6 in, 1 out]
                        }
                        frame "MIN" {
                          n177 = call "MLLF_FormatStringValue.vi"("error in"=w695, "String Value"=w692, "Format"="BAND MIN" ("format string")) -> ("error out"=w696:T15, "String Value Formated"=w694:T16)  [unwired: 6 in, 1 out]
                        }
                      }
                      n178 = Search and Replace String(replace all?=w663, case sensitive?=w663, input string=w665, search string="\"") -> (result string=w664:string)  [unwired: 4 in, 3 out]
                      n179 = Match Pattern(string=w664, regular expression="[\\s\\t]+") -> (before substring=w666:string)  [unwired: 1 in, 3 out]
                      n180 = Concatenate Strings(w666, ":" ("string"), w668) -> (w661:string)
                      n181 = call "MLLF_WriteToBuffer.vi"("String"=w661, "error in"=w681, "DriverConnect in"=w670) -> ("error out"=w680:T15, "DriverConnect out"=w679:T1)  [unwired: 5 in]
                      n182 = call "AgilentDMM_ESR_check.vi"("Driver Name"=w676, "Error Code"=w677, "Model"=w659, "error in"=w680, "DriverConnect in"=w679) -> ("error out"=w678:T15)  [unwired: 5 in, 1 out]
                    }
                    frame "34401" {
                      w702 = TRUE ("replace all? (F)")
                      n183 = call "MLLF_WriteToBuffer.vi"("String"="CONFigure? ", "DriverConnect in"=w712) -> ("error out"=w709:T15, "DriverConnect out"=w710:T1)  [unwired: 6 in]
                      n184 = call "MLLF_ReadBuffer.vi"("Error In"=w709, "DriverConnect in"=w710) -> ("Error Out"=w708:errorcluster, "DriverConnect out"=w707:T1, "String"=w704:string)  [unwired: 6 in]
                      n185 = case shown="\"MAX\"" w699 {
                        tunnel: [w723 w728 w733] -> w718
                        tunnel: w708 -> [w722 w727 w732]
                        tunnel: [w721 w726 w731] -> w705
                        tunnel: w699 -> [w719 w724 w729]
                        frame Default {
                          n186 = call "MLLF_FormatStringValue.vi"("error in"=w722, "String Value"=w719, "Format"="BAND %#f" ("format string")) -> ("error out"=w723:T15, "String Value Formated"=w721:T16)  [unwired: 6 in, 1 out]
                        }
                        frame "MAX" {
                          n187 = call "MLLF_FormatStringValue.vi"("error in"=w727, "String Value"=w724, "Format"="BAND MAX" ("format string")) -> ("error out"=w728:T15, "String Value Formated"=w726:T16)  [unwired: 6 in, 1 out]
                        }
                        frame "MIN" {
                          n188 = call "MLLF_FormatStringValue.vi"("error in"=w732, "String Value"=w729, "Format"="BAND MIN" ("format string")) -> ("error out"=w733:T15, "String Value Formated"=w731:T16)  [unwired: 6 in, 1 out]
                        }
                      }
                      n189 = Search and Replace String(replace all?=w702, case sensitive?=w702, input string=w704, search string="\"") -> (result string=w703:string)  [unwired: 4 in, 3 out]
                      n190 = Match Pattern(string=w703, regular expression="[\\s\\t]+") -> ()  [unwired: 1 in, 4 out]
                      n191 = Concatenate Strings(":DET:" ("string"), w705) -> (w700:string)
                      n192 = call "MLLF_WriteToBuffer.vi"("String"=w700, "error in"=w718, "DriverConnect in"=w707) -> ("error out"=w717:T15, "DriverConnect out"=w716:T1)  [unwired: 5 in]
                      n193 = call "AgilentDMM_ESR_check.vi"("Driver Name"=w713, "Error Code"=w714, "Model"=w697, "error in"=w717, "DriverConnect in"=w716) -> ("error out"=w715:T15)  [unwired: 5 in, 1 out]
                    }
                  }
                }
                frame "AutoZero", "ZERO" {
                  n194 = case shown="\"34461\", Default" w734 {
                    tunnel: [w765 w793] -> w740
                    tunnel: w734 -> [w764 w792]
                    tunnel: w739 -> [w763 w791]
                    tunnel: w738 -> [w748 w776]
                    tunnel: w737 -> [w747 w775]
                    tunnel: w736 -> [w743 w771]
                    tunnel: w735 -> [w742 w770]
                    frame "34461", Default {
                      w753 = TRUE ("replace all? (F)")
                      n195 = call "MLLF_WriteToBuffer.vi"("String"="CONFigure? ", "DriverConnect in"=w763) -> ("error out"=w760:T15, "DriverConnect out"=w761:T1)  [unwired: 6 in]
                      n196 = call "MLLF_ReadBuffer.vi"("Error In"=w760, "DriverConnect in"=w761) -> ("Error Out"=w745:errorcluster, "DriverConnect out"=w759:T1, "String"=w755:string)  [unwired: 6 in]
                      n197 = Search and Replace String(replace all?=w753, case sensitive?=w753, input string=w755, search string="\"") -> (result string=w754:string)  [unwired: 4 in, 3 out]
                      n198 = Match Pattern(string=w754, regular expression="[\\s\\t]+") -> (before substring=w756:string)  [unwired: 1 in, 3 out]
                      n199 = call "MLLF_ParameterSelect.vi"("Command to equipment"=string[] ["ZERO:AUTO OFF", "ZERO:AUTO ON", "ZERO:AUTO ONCE"] ("Names"), "Names"=string[][] [["0", "DIS", "DISABLE", "DISABLED", "OFF"], ["1", "EN", "ENABLE", "ENABLED", "ON"], [" ", "", "", "", ""]], "Input"=w743, "Error In"=w745, "Command"=w742, "Driver Name"=w748, "Error Code"=w747) -> ("Choice"=w744:string, "Error Out"=w746:errorcluster)  [unwired: 7 in]
                      n200 = Concatenate Strings(w756, ":" ("string"), w744) -> (w751:string)
                      n201 = call "MLLF_WriteToBuffer.vi"("String"=w751, "error in"=w746, "DriverConnect in"=w759) -> ("error out"=w767:T15, "DriverConnect out"=w766:T1)  [unwired: 5 in]
                      n202 = call "AgilentDMM_ESR_check.vi"("Driver Name"=w748, "Error Code"=w747, "Model"=w764, "error in"=w767, "DriverConnect in"=w766) -> ("error out"=w765:T15)  [unwired: 5 in, 1 out]
                    }
                    frame "34401" {
                      w781 = TRUE ("replace all? (F)")
                      n203 = call "MLLF_WriteToBuffer.vi"("String"="CONFigure? ", "DriverConnect in"=w791) -> ("error out"=w788:T15, "DriverConnect out"=w789:T1)  [unwired: 6 in]
                      n204 = call "MLLF_ReadBuffer.vi"("Error In"=w788, "DriverConnect in"=w789) -> ("Error Out"=w773:errorcluster, "DriverConnect out"=w787:T1, "String"=w783:string)  [unwired: 6 in]
                      n205 = Search and Replace String(replace all?=w781, case sensitive?=w781, input string=w783, search string="\"") -> (result string=w782:string)  [unwired: 4 in, 3 out]
                      n206 = Match Pattern(string=w782, regular expression="[\\s\\t]+") -> (before substring=w784:string)  [unwired: 1 in, 3 out]
                      n207 = call "MLLF_ParameterSelect.vi"("Command to equipment"=string[] ["ZERO:AUTO OFF", "ZERO:AUTO ON", "ZERO:AUTO ONCE"] ("Names"), "Ignor case(default = true)"=TRUE, "Names"=string[][] [["OFF"], ["ON"], ["ONCE"]], "Input"=w771, "Error In"=w773, "Command"=w770, "Driver Name"=w776, "Error Code"=w775) -> ("Choice"=w772:string, "Error Out"=w774:errorcluster)  [unwired: 6 in]
                      n208 = Concatenate Strings("SENSe:" ("string"), w784, ":" ("string"), w772) -> (w779:string)
                      n209 = call "MLLF_WriteToBuffer.vi"("String"=w779, "error in"=w774, "DriverConnect in"=w787) -> ("error out"=w795:T15, "DriverConnect out"=w794:T1)  [unwired: 5 in]
                      n210 = call "AgilentDMM_ESR_check.vi"("Driver Name"=w776, "Error Code"=w775, "Model"=w792, "error in"=w795, "DriverConnect in"=w794) -> ("error out"=w793:T15)  [unwired: 5 in, 1 out]
                    }
                  }
                }
                frame "LOWPOWER" {
                  w807 = TRUE ("replace all? (F)")
                  n211 = call "MLLF_WriteToBuffer.vi"("String"="CONFigure? ", "DriverConnect in"=w817) -> ("error out"=w814:T15, "DriverConnect out"=w815:T1)  [unwired: 6 in]
                  n212 = call "MLLF_ReadBuffer.vi"("Error In"=w814, "DriverConnect in"=w815) -> ("Error Out"=w799:errorcluster, "DriverConnect out"=w813:T1, "String"=w809:string)  [unwired: 6 in]
                  n213 = Search and Replace String(replace all?=w807, case sensitive?=w807, input string=w809, search string="\"") -> (result string=w808:string)  [unwired: 4 in, 3 out]
                  n214 = Match Pattern(string=w808, regular expression="[\\s\\t]+") -> (before substring=w810:string)  [unwired: 1 in, 3 out]
                  n215 = call "MLLF_ParameterSelect.vi"("Command to equipment"=string[] ["POW:LIM OFF", "POW:LIM ON"] ("Names"), "Names"=string[][] [["0", "DIS", "DISABLE", "DISABLED", "OFF"], ["1", "EN", "ENABLE", "ENABLED", "ON"]], "Input"=w797, "Error In"=w799, "Command"=w796, "Driver Name"=w802, "Error Code"=w801) -> ("Choice"=w798:string, "Error Out"=w800:errorcluster)  [unwired: 7 in]
                  n216 = Concatenate Strings(w810, ":" ("string"), w798) -> (w805:string)
                  n217 = call "MLLF_WriteToBuffer.vi"("String"=w805, "error in"=w800, "DriverConnect in"=w813) -> ("error out"=w822:T15, "DriverConnect out"=w821:T1)  [unwired: 5 in]
                  n218 = call "AgilentDMM_ESR_check.vi"("Driver Name"=w802, "Error Code"=w801, "Model"=w818, "error in"=w822, "DriverConnect in"=w821) -> ("error out"=w819:T15)  [unwired: 5 in, 1 out]
                }
                frame "VOLTAGELIMITED" {
                  w834 = TRUE ("replace all? (F)")
                  n219 = call "MLLF_WriteToBuffer.vi"("String"="CONFigure? ", "DriverConnect in"=w844) -> ("error out"=w841:T15, "DriverConnect out"=w842:T1)  [unwired: 6 in]
                  n220 = call "MLLF_ReadBuffer.vi"("Error In"=w841, "DriverConnect in"=w842) -> ("Error Out"=w826:errorcluster, "DriverConnect out"=w840:T1, "String"=w836:string)  [unwired: 6 in]
                  n221 = Search and Replace String(replace all?=w834, case sensitive?=w834, input string=w836, search string="\"") -> (result string=w835:string)  [unwired: 4 in, 3 out]
                  n222 = Match Pattern(string=w835, regular expression="[\\s\\t]+") -> (before substring=w837:string)  [unwired: 1 in, 3 out]
                  n223 = call "MLLF_ParameterSelect.vi"("Command to equipment"=string[] ["VOLT:LIM OFF", "VOLT:LIM ON"] ("Names"), "Names"=string[][] [["0", "DIS", "DISABLE", "DISABLED", "OFF"], ["1", "EN", "ENABLE", "ENABLED", "ON"]], "Input"=w824, "Error In"=w826, "Command"=w823, "Driver Name"=w829, "Error Code"=w828) -> ("Choice"=w825:string, "Error Out"=w827:errorcluster)  [unwired: 7 in]
                  n224 = Concatenate Strings(w837, ":" ("string"), w825) -> (w832:string)
                  n225 = call "MLLF_WriteToBuffer.vi"("String"=w832, "error in"=w827, "DriverConnect in"=w840) -> ("error out"=w849:T15, "DriverConnect out"=w848:T1)  [unwired: 5 in]
                  n226 = call "AgilentDMM_ESR_check.vi"("Driver Name"=w829, "Error Code"=w828, "Model"=w845, "error in"=w849, "DriverConnect in"=w848) -> ("error out"=w846:T15)  [unwired: 5 in, 1 out]
                }
                frame "FILT", "FILTER" {
                  # "FILT=DIS"
                  n227 = call "MLLF_ParameterSelect.vi"("Command to equipment"=string[] ["INPut:FILTer:STATE OFF", "INPut:FILTer:STATE ON"] ("Names"), "Names"=string[][] [["0", "DIS", "DISABLE", "DISABLED", "OFF"], ["1", "EN", "ENABLE", "ENABLED", "ON"]], "Input"=w851, "Command"=w850, "Driver Name"=w856, "Error Code"=w855) -> ("Choice"=w852:string, "Error Out"=w854:errorcluster)  [unwired: 8 in]
                  n228 = call "MLLF_WriteToBuffer.vi"("String"=w852, "error in"=w854, "DriverConnect in"=w853) -> ("error out"=w863:T15, "DriverConnect out"=w862:T1)  [unwired: 5 in]
                  n229 = call "AgilentDMM_ESR_check.vi"("Driver Name"=w856, "Error Code"=w855, "Model"=w859, "error in"=w863, "DriverConnect in"=w862) -> ("error out"=w860:T15)  [unwired: 5 in, 1 out]
                }
                frame "SND", "Sound" {
                  # "sound"
                  # "sound=off"
                  n230 = call "MLLF_ParameterSelect.vi"("Command to equipment"=string[] ["SYST:BEEP:STAT OFF", "SYST:BEEP:STAT ON", "SYST:BEEP"] ("Names"), "Names"=string[][] [["0", "DIS", "DISABLED", "DISABLE", "OFF"], ["1", "EN", "ENABLE", "ENABLED", "ON"], [" ", "", "", "", ""]], "Input"=w865, "Command"=w864, "Driver Name"=w872, "Error Code"=w873) -> ("Choice"=w868:string, "Error Out"=w870:errorcluster)  [unwired: 8 in]
                  n231 = call "MLLF_WriteToBuffer.vi"("String"=w868, "error in"=w870, "DriverConnect in"=w869) -> ("error out"=w875:T15, "DriverConnect out"=w874:T1)  [unwired: 5 in]
                  n232 = call "AgilentDMM_ESR_check.vi"("Driver Name"=w872, "Error Code"=w873, "Model"=w876, "error in"=w875, "DriverConnect in"=w874) -> ("error out"=w871:T15)  [unwired: 5 in, 1 out]
                }
              }
            }
            frame #2 {
            }
          }
        }
        frame "get" {
          n233 = flat-sequence {
            tunnel: w899 -> [w910]
            tunnel: w900 -> [w911]
            tunnel: w901 -> [w912]
            tunnel: w889 -> [w903]
            tunnel: [w903] -> w898
            tunnel: [w912] -> w897
            tunnel: [w911] -> w896
            tunnel: [w908] -> w895
            tunnel: [w909] -> w894
            tunnel: [w907] -> w893
            tunnel: [w904] -> w892
            tunnel: [w905] -> w891
            tunnel: [w910] -> w890
            tunnel: w888 -> [w906]
            tunnel: w898 -> [w926]
            tunnel: w897 -> [w924]
            tunnel: w896 -> [w923]
            tunnel: w895 -> [w920]
            tunnel: w894 -> [w919]
            tunnel: w893 -> [w918]
            tunnel: w892 -> [w917]
            tunnel: w891 -> [w916]
            tunnel: w890 -> [w913]
            tunnel: [w925] -> w887
            tunnel: [w922] -> w886
            tunnel: [w921] -> w885
            tunnel: [w915] -> w884
            tunnel: [w914] -> w883
            tunnel: [w1065] -> w902
            tunnel: w887 -> [w1065]
            tunnel: w886 -> [w1063]
            tunnel: w885 -> [w1062]
            tunnel: w884 -> [w1064]
            tunnel: w883 -> [w1061]
            tunnel: [w1060] -> w882
            tunnel: [w1059] -> w881
            frame #0 {
              n234 = Unbundle By Name(w903) -> ("Data.Model"=w909:T8, "Data.Connect"=w908:T1, "Data.Func"=w907:T7)
              n235 = call "MLLF_CommandDelimeter.vi"("command with param"=w906) -> ("param 1"=w905:string, "command"=w904:string)  [unwired: 6 in, 3 out]
            }
            frame #1 {
              n236 = case shown="\"CONF\", \"CONFIG\", \"CONFIGURATION\"" w917 {
                selector: w917 -> [w928 _ _ _ _ _ _]
                tunnel: [w927 w932 w946 w978 w993 w1019 w1045] -> w922
                tunnel: w924 -> [_ _ w939 w977 w986 w1012 w1039]
                tunnel: [w931 w935 w948 w980 w995 w1021 w1047] -> w925
                tunnel: w926 -> [w931 w935 w948 w980 w995 w1021 w1047]
                tunnel: [w929 w933 w941 _ w988 w1014 _] -> w921
                tunnel: w920 -> [_ _ w947 w979 w994 w1020 w1046]
                tunnel: w923 -> [_ _ w938 w976 w985 w1011 w1038]
                tunnel: w916 -> [_ _ w942 w968 w989 w1015 w1041]
                tunnel: w919 -> [_ _ w937 w975 w984 w1010 w1037]
                tunnel: w918 -> [_ _ w936 w974 w983 _ _]
                tunnel: [_ _ _ TRUE ("use system decimal point (T)") _ _ TRUE ("use system decimal point (T)")] -> w915
                tunnel: [_ _ _ w966 _ _ w1035] -> w914
                tunnel: w913 -> [_ w932 _ _ _ _ _]
                frame "False", Default {
                  n237 = call "MLLF_UnknownCommand(SubVI).vi"("Unknown command"=w928) -> ("error out"=w927:errorcluster)  [unwired: 10 in]
                  n238 = Build Array(0.0 ("TimeOut")) -> (w929:dbl[])
                }
                frame "TIMEOUT" {
                  n239 = Unbundle By Name(w935) -> ("Data.Connect.InterfaceSettings.TMO, ms"=w934:i32)
                  n240 = Build Array(w934) -> (w933:i32[])
                }
                frame "READ" {
                  n241 = Decimal String To Number(string=w942) -> (number=w943:i32)  [unwired: 2 in, 1 out]
                  n242 = In Range and Coerce(upper limit=100, x=w943, lower limit=1) -> (coerced(x)=w940:i32)  [unwired: 1 out]
                  n243 = for {
                    N: w940 -> [_]
                    tunnel: [w960] -> w941 mode=indexing
                    tunnel: w947 -> [w959]
                    tunnel: [w954] -> w946
                    tunnel: w939 -> [w953]
                    tunnel: w938 -> [w952]
                    tunnel: w937 -> [w951]
                    tunnel: w936 -> [w949]
                    stop <- w954 stop-if-true
                    n244 = case shown="\"VDC\", Default" w949 {
                      tunnel: [1.0 ("Delay Time (s)") 0.05 ("Delay Time (s)")] -> w950
                      frame "F" {
                      }
                      frame "VDC", Default {
                      }
                    }
                    n245 = call "MLLF_WriteToBufferWithDelay.vi"("Delay Time ( 0,05 s)"=w950, "Command"="READ? " ("String"), "DriverConnect in"=w959) -> ("Error Out"=w963:errorcluster, "DriverConnect out"=w962:T1)  [unwired: 7 in]
                    n246 = call "MLLF_ReadBuffer.vi"("Error In"=w963, "DriverConnect in"=w962) -> ("Error Out"=w956:errorcluster, "DriverConnect out"=w955:T1, "String"=w958:string)  [unwired: 6 in]
                    n247 = call "AgilentDMM_ESR_check.vi"("Driver Name"=w952, "Error Code"=w953, "Model"=w951, "error in"=w956, "DriverConnect in"=w955) -> ("error out"=w954:T15)  [unwired: 5 in, 1 out]
                    n248 = Fract/Exp String To Number(use system decimal point (T)=FALSE, string=w958) -> (number=w960:dbl)  [unwired: 2 in, 1 out]
                  }
                }
                frame "SCPI" {
                  n249 = case shown="\"VDC\", Default" w974 {
                    tunnel: [1.0 ("Delay Time (s)") 0.05 ("Delay Time (s)")] -> w969
                    frame "F" {
                    }
                    frame "VDC", Default {
                    }
                  }
                  n250 = call "MLLF_WriteToBufferWithDelay.vi"("Delay Time ( 0,05 s)"=w969, "Command"=w968, "DriverConnect in"=w979) -> ("Error Out"=w973:errorcluster, "DriverConnect out"=w972:T1)  [unwired: 7 in]
                  n251 = call "MLLF_ReadBuffer.vi"("Error In"=w973, "DriverConnect in"=w972) -> ("Error Out"=w971:errorcluster, "DriverConnect out"=w970:T1, "String"=w966:string)  [unwired: 6 in]
                  n252 = call "AgilentDMM_ESR_check.vi"("Driver Name"=w976, "Error Code"=w977, "Model"=w975, "error in"=w971, "DriverConnect in"=w970) -> ("error out"=w978:T15)  [unwired: 5 in, 1 out]
                }
                frame "SelfTest" {
                  n253 = Decimal String To Number(string=w989) -> (number=w990:i32)  [unwired: 2 in, 1 out]
                  n254 = In Range and Coerce(upper limit=100, x=w990, lower limit=1) -> (coerced(x)=w987:i32)  [unwired: 1 out]
                  n255 = for {
                    N: w987 -> [_]
                    tunnel: [w1007] -> w988 mode=indexing
                    tunnel: w994 -> [w1006]
                    tunnel: [w1001] -> w993
                    tunnel: w986 -> [w1000]
                    tunnel: w985 -> [w999]
                    tunnel: w984 -> [w998]
                    tunnel: w983 -> [_]
                    stop <- w1001 stop-if-true
                    n256 = call "MLLF_WriteToBufferWithDelay.vi"("Command"="*TST? " ("String"), "DriverConnect in"=w1006) -> ("Error Out"=w997:errorcluster, "DriverConnect out"=w1009:T1)  [unwired: 8 in]
                    n257 = call "Time Delay"("error in (no error)"=w997) -> ("error out"=w996:errorcluster)  [unwired: 10 in]
                    n258 = call "MLLF_ReadBuffer.vi"("Error In"=w996, "DriverConnect in"=w1009) -> ("Error Out"=w1003:errorcluster, "DriverConnect out"=w1002:T1, "String"=w1005:string)  [unwired: 6 in]
                    n259 = call "AgilentDMM_ESR_check.vi"("Driver Name"=w999, "Error Code"=w1000, "Model"=w998, "error in"=w1003, "DriverConnect in"=w1002) -> ("error out"=w1001:T15)  [unwired: 5 in, 1 out]
                    n260 = Fract/Exp String To Number(use system decimal point (T)=FALSE, string=w1005) -> (number=w1007:dbl)  [unwired: 2 in, 1 out]
                  }
                }
                frame "FETCH" {
                  n261 = Decimal String To Number(string=w1015) -> (number=w1016:i32)  [unwired: 2 in, 1 out]
                  n262 = In Range and Coerce(upper limit=100, x=w1016, lower limit=1) -> (coerced(x)=w1013:i32)  [unwired: 1 out]
                  n263 = for {
                    N: w1013 -> [_]
                    tunnel: [w1031] -> w1014 mode=indexing
                    tunnel: w1020 -> [w1030]
                    tunnel: [w1025] -> w1019
                    tunnel: w1012 -> [w1024]
                    tunnel: w1011 -> [w1023]
                    tunnel: w1010 -> [w1022]
                    stop <- w1025 stop-if-true
                    n264 = call "MLLF_WriteToBuffer.vi"("String"="FETC? ", "DriverConnect in"=w1030) -> ("error out"=w1034:T15, "DriverConnect out"=w1033:T1)  [unwired: 6 in]
                    n265 = call "MLLF_ReadBuffer.vi"("Error In"=w1034, "DriverConnect in"=w1033) -> ("Error Out"=w1027:errorcluster, "DriverConnect out"=w1026:T1, "String"=w1029:string)  [unwired: 6 in]
                    n266 = call "AgilentDMM_ESR_check.vi"("Driver Name"=w1023, "Error Code"=w1024, "Model"=w1022, "error in"=w1027, "DriverConnect in"=w1026) -> ("error out"=w1025:T15)  [unwired: 5 in, 1 out]
                    n267 = Fract/Exp String To Number(use system decimal point (T)=FALSE, string=w1029) -> (number=w1031:dbl)  [unwired: 2 in, 1 out]
                  }
                }
                frame "CONF", "CONFIG", "CONFIGURATION" {
                  n268 = Decimal String To Number(string=w1041) -> (number=w1042:i32)  [unwired: 2 in, 1 out]
                  n269 = In Range and Coerce(upper limit=100, x=w1042, lower limit=1) -> (coerced(x)=w1040:i32)  [unwired: 1 out]
                  n270 = for {
                    N: w1040 -> [_]
                    tunnel: w1046 -> [w1056]
                    tunnel: [w1052] -> w1045
                    tunnel: w1039 -> [w1051]
                    tunnel: w1038 -> [w1050]
                    tunnel: w1037 -> [w1049]
                    tunnel: [w1048] -> w1035
                    stop <- w1052 stop-if-true
                    n271 = call "MLLF_WriteToBuffer.vi"("String"="CONFigure? ", "DriverConnect in"=w1056) -> ("error out"=w1058:T15, "DriverConnect out"=w1057:T1)  [unwired: 6 in]
                    n272 = call "MLLF_ReadBuffer.vi"("Error In"=w1058, "DriverConnect in"=w1057) -> ("Error Out"=w1054:errorcluster, "DriverConnect out"=w1053:T1, "String"=w1048:string)  [unwired: 6 in]
                    n273 = call "AgilentDMM_ESR_check.vi"("Driver Name"=w1050, "Error Code"=w1051, "Model"=w1049, "error in"=w1054, "DriverConnect in"=w1053) -> ("error out"=w1052:T15)  [unwired: 5 in, 1 out]
                  }
                }
              }
            }
            frame #2 {
              n274 = case shown="False" w1064 {
                tunnel: w1063 -> [w1070 w1071]
                tunnel: w1062 -> [w1069 _]
                tunnel: [w1067 w1071] -> w1060
                tunnel: [w1066 w1072] -> w1059
                tunnel: w1061 -> [_ w1072]
                frame False {
                  n275 = call "MLLF_FormatOutputValueWithUnits.vi"("Format"="%.;%^#_8e" ("format string"), "error in"=w1070, "ValuesIn"=w1069) -> ("error out"=w1067:T15, "Result string"=w1066:T16)  [unwired: 7 in]
                }
                frame True {
                }
              }
            }
          }
        }
        frame "close" {
          n276 = Unbundle By Name(w1074) -> ("Data.Connect.OpenedSession"=w1076:T3)
          n277 = VISA Close(VISA resource name=w1076) -> (error out=w1075:errorcluster)  [unwired: 1 in]
        }
      }
    }
    frame Error {
    }
  }
  n278 = local write "Settings"(w1) -> ()
  n279 = flat-sequence {
    tunnel: [w1088] -> w2
    tunnel: [w1087] -> w4
    tunnel: w7 -> [w1086]
    tunnel: w5 -> [w1085]
    tunnel: w6 -> [w1081]
    tunnel: [w1083] -> w3
    frame #0 {
      # "driver out"
      n280 = Unbundle By Name(w1081) -> ("Data"=w1080:T17)
      n281 = To Variant(anything=w1080) -> (Variant=w1082:variant)
      n282 = Bundle By Name(cluster=w1081, "Saved Data"=w1082) -> (w1083:T9)
      n283 = call "MLLF_SaveLastSettingUtility.vi"("error in"=w1085, "Saved Data"=w1082) -> ("error out"=w1084:T15)  [unwired: 8 in, 1 out]
      n284 = call "MCF_Output.vi"("Error In"=w1084, "Input"=w1086) -> ("Error Out"=w1087:errorcluster, "Output"=w1088:string)  [unwired: 8 in]
    }
  }
  n285 = local write "Settings"(w3) -> ()
  "error out" <- w4
  "Response" <- w2
